vi "Update cursor position.vi"(8 "error in (no error)":errorcluster, 9 "Position Y":dbl, 10 "index":i32, 11 "LIVE DATA 3":refnum<vi>) -> (0 "error out":errorcluster)   [LabVIEW 2016]
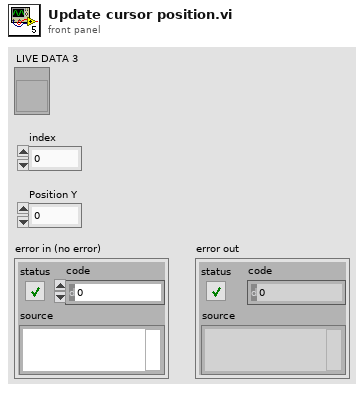
[diagram p1: front panel]
types:
  T1 = typedef "LVCursorListTypeDef.ctl" = cluster{"Name":string, "Color":u32, "Style":u8, "Point Style":u8, "Name Visible":bool, "Allow Drag":bool, "Cursor Mode":u32, "Plot":i32, "Index":i32, "Position":cluster{"X":dbl, "Y":dbl}, "X Scale":u32, "Y Scale":u32, "Watch Plots":i32[], "Watch All Plots":bool, "Plot Area":i32, "Label Offset":cluster{"X":dbl, "Y":dbl}}[]
  T2 = cluster{"Name":string, "Color":u32, "Style":u8, "Point Style":u8, "Name Visible":bool, "Allow Drag":bool, "Cursor Mode":u32, "Plot":i32, "Index":i32, "Position":cluster{"X":dbl, "Y":dbl}, "X Scale":u32, "Y Scale":u32, "Watch Plots":i32[], "Watch All Plots":bool, "Plot Area":i32, "Label Offset":cluster{"X":dbl, "Y":dbl}}
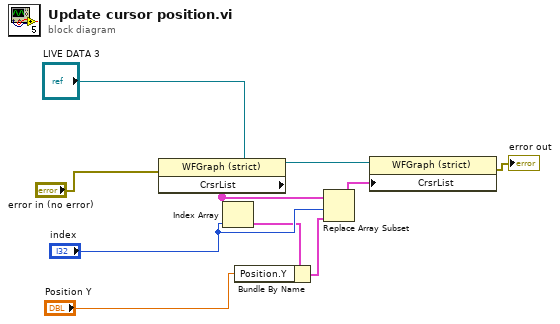
[diagram p0: block diagram]
diagram:
  n1 = property class="WFGraph (strict)"(reference="LIVE DATA 3", error in="error in (no error)") -> (reference out=w8:refnum<vi>, "CrsrList"=w5:T1)  [unwired: 1 out]
  n2 = Index Array(array=w5, index="index") -> (element=w4:T2)
  n3 = Bundle By Name(cluster=w4, "Position.Y"="Position Y") -> (w7:T2)
  n4 = Replace Array Subset(array=w5, new element=w7, index="index") -> (w9:T1)
  n5 = property class="WFGraph (strict)"(reference=w8, "CrsrList"=w9) -> (error out=→"error out":errorcluster)  [unwired: 1 in, 1 out]
